vi "Connection_Management.vi"(0 "CM Packet In":T3, 5 "Commands":T7, 7 "Retry interval (ms)":i32, 9 "Number of tries":u8, 11 "error in (no error)":errorcluster) -> (4 "CM Packet Out":T3, 6 "CM Params Out":T2, 8 "Network Error Status":T1(ring), 15 "error out":errorcluster)   [LabVIEW 2017]
uses:
  Controls/Packet/Packet.ctl
  Controls/Packet/Packet_Direction.ctl
  Controls/Packet/Packet_Type.ctl
  Controls/Packet/Packet_Priority.ctl
  Controls/Connection Management/Connection_Management_Commands.ctl
  Controls/Control Packets/CM_Param.ctl
  <vilib>/Instr/_visa.llb/VISA Flush IO Buffer Mask.ctl
panel:
  out "Try counter (SYNC/RST)":i32
  out "Try counter (CC)":i32
  out "Try counter (OC)":i32
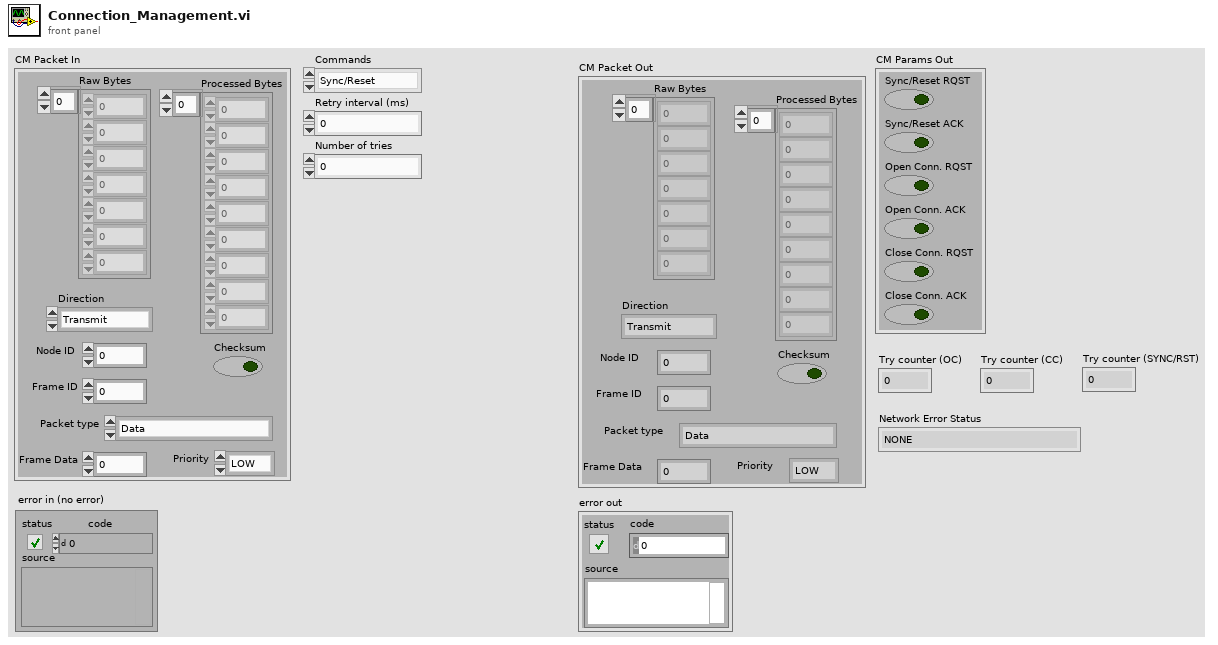
[diagram p1: front panel]
types:
  T1 = enum16{"NONE", "CONNECTION_ALREADY_OPEN", "CONNECTION_ALREADY_CLOSED", "INVALID_FRAME_REQUEST"}
  T2 = typedef "CM_Param.ctl" = cluster{"Sync/Reset RQST":bool, "Sync/Reset ACK":bool, "Open Conn. RQST":bool, "Open Conn. ACK":bool, "Close Conn. RQST":bool, "Close Conn. ACK":bool}
  T3 = typedef "Packet.ctl" = cluster{"Raw Bytes":u8[], "Checksum":bool, "Direction":T4, "Processed Bytes":u8[], "Node ID":u8, "Packet type":T5, "Frame Data":u32, "Priority":T6, "Frame ID":u8}
  T4 = typedef "Packet_Direction.ctl" = enum16{"Transmit", "Receive", "Bidirectional"}
  T5 = typedef "Packet_Type.ctl" = enum16{"Data", "Connection Management", "Remote Request", "Error/Status"}
  T6 = typedef "Packet_Priority.ctl" = enum16{"LOW", "HIGH"}
  T7 = typedef "Connection_Management_Commands.ctl" = enum16{"Sync/Reset", "Open Connection", "Close Connection"}
  T8 = typedef "VISA Flush IO Buffer Mask.ctl" = u16
  T9 = typedef "ES_Param.ctl" = cluster{"Status Request":bool, "Status Ack.":bool, "Receiver Queue Status":enum16{"OK", "EMPTY", "FULL"}, "Network Error Status":enum16{"NONE", "CONNECTION_ALREADY_OPEN", "CONNECTION_ALREADY_CLOSED", "INVALID_FRAME_REQUEST"}, "Application Error Code":u16, "Receiver Queue Size":i32}
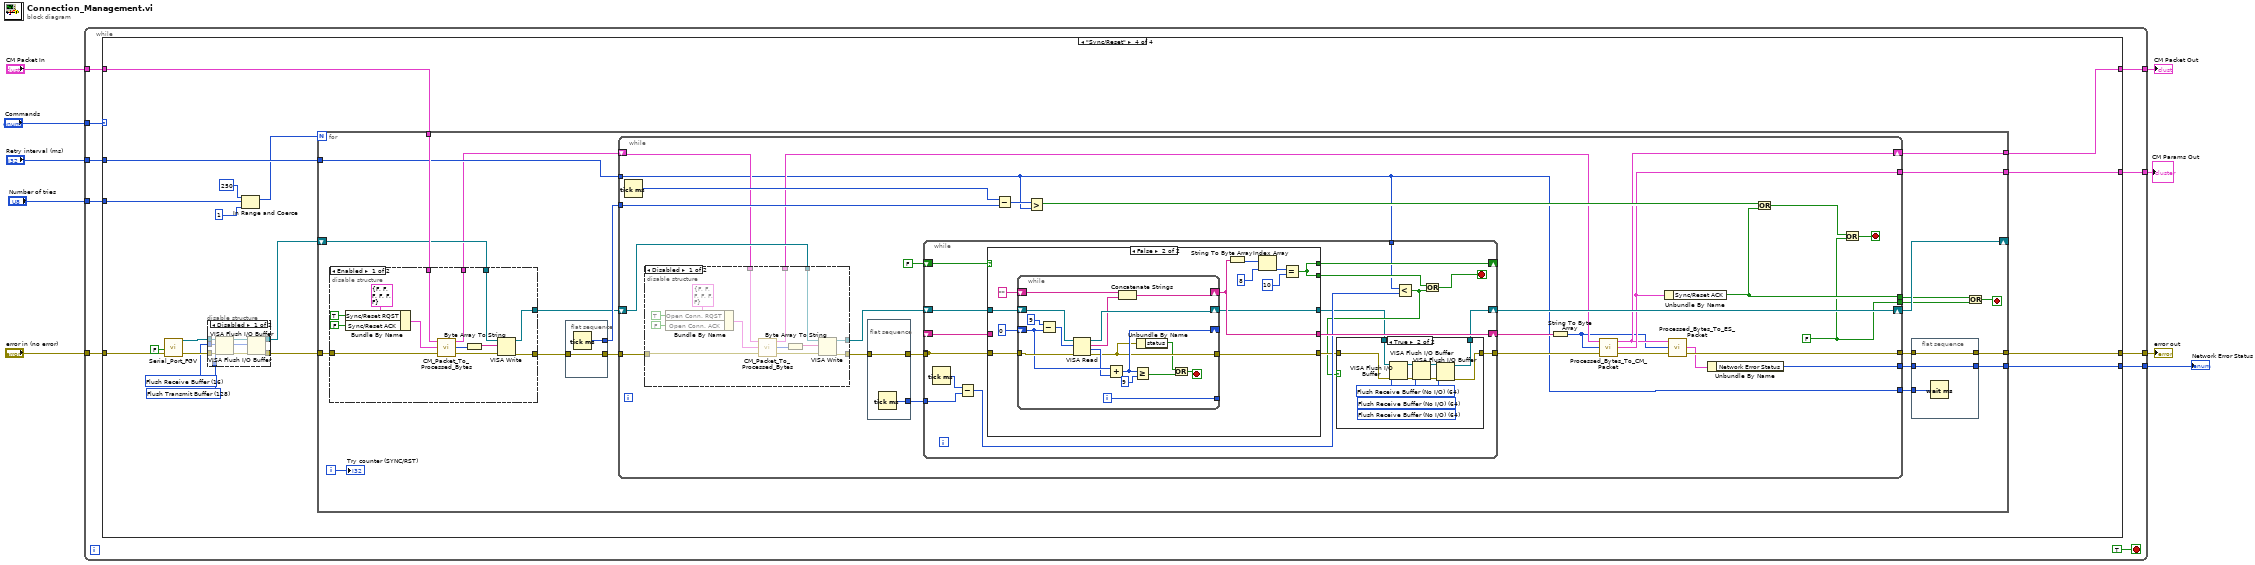
[diagram p0: block diagram]
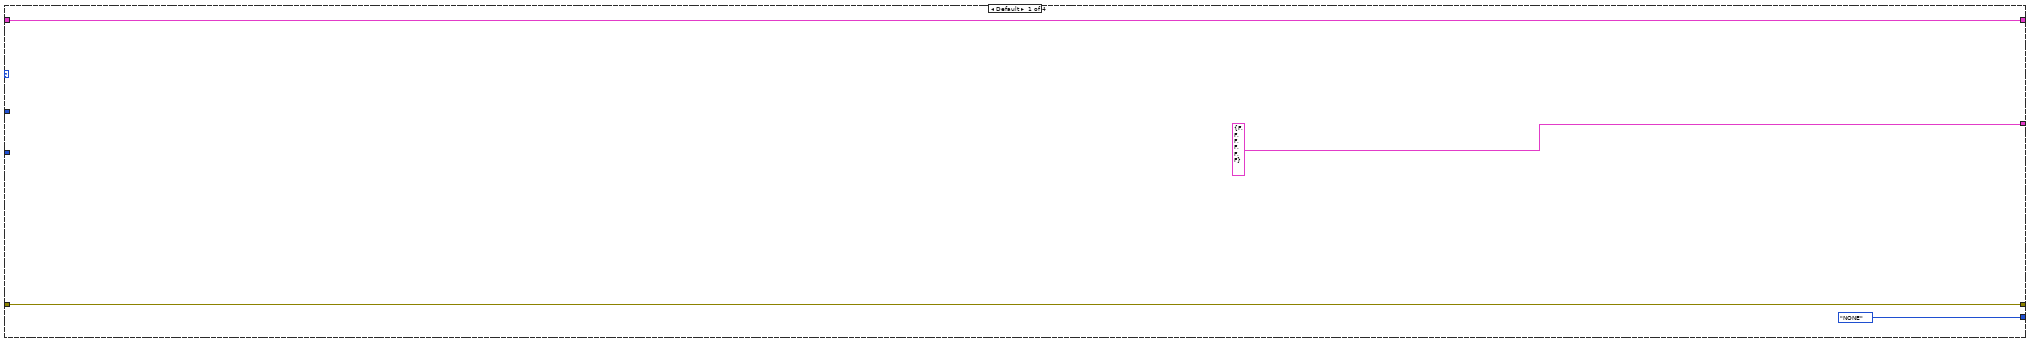
[diagram p2: hidden frame]
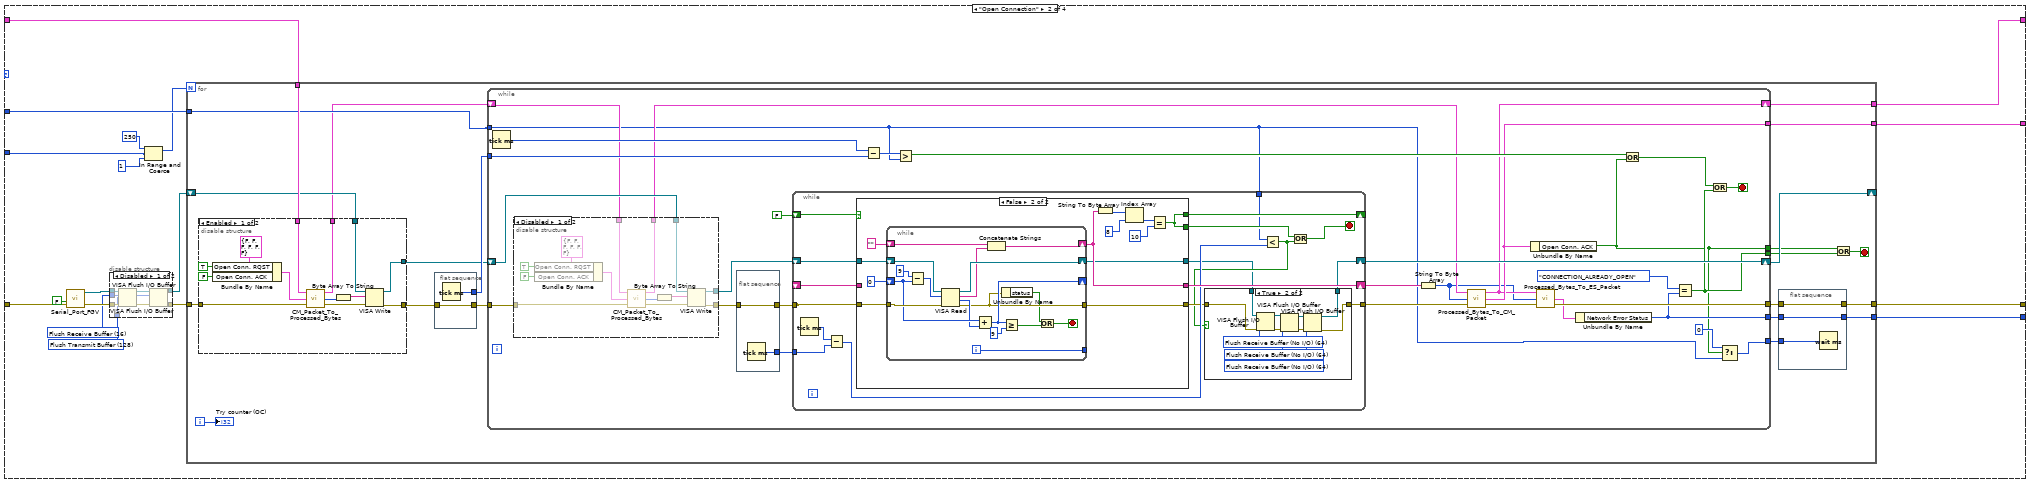
[diagram p3: hidden frame]
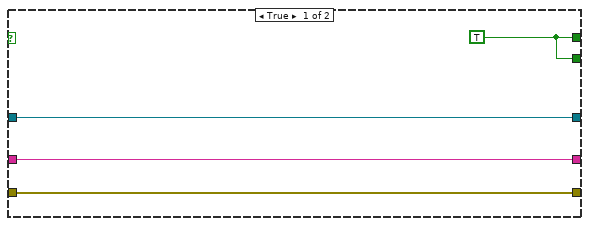
[diagram p8: hidden frame]
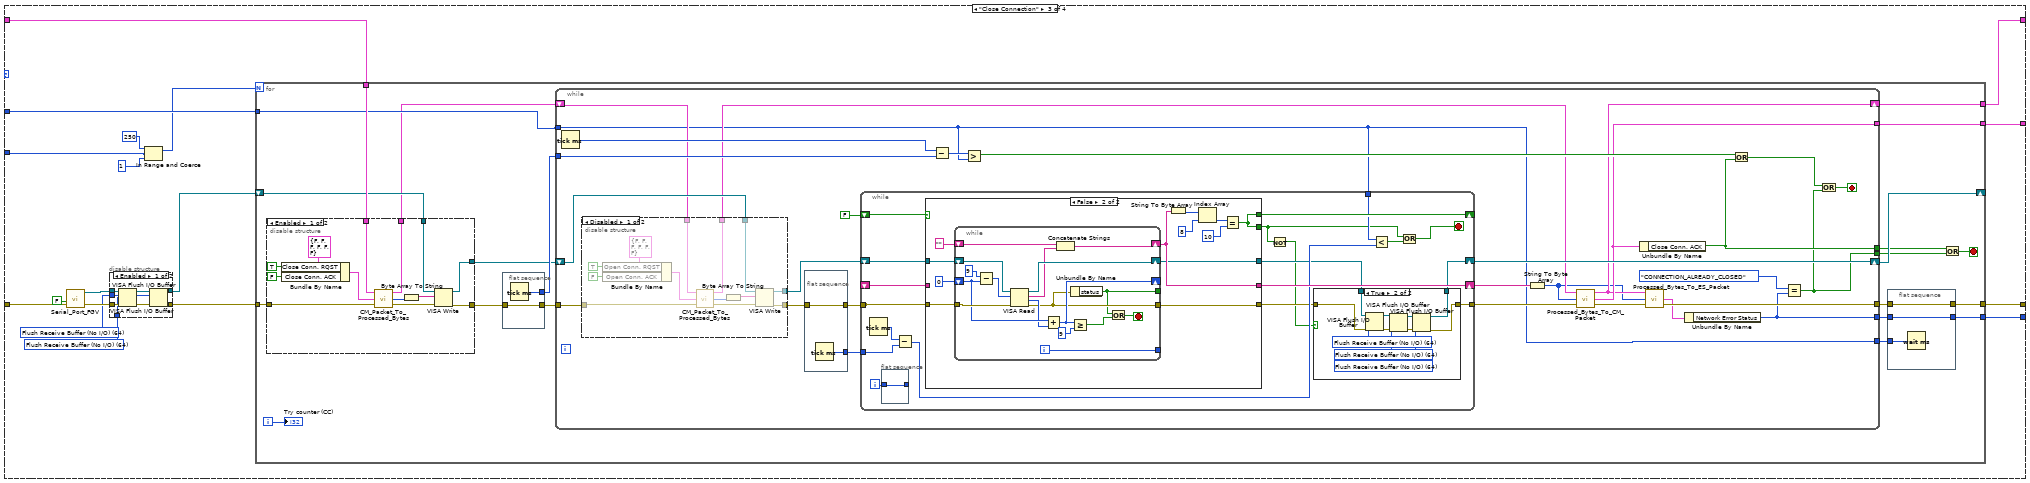
[diagram p9: hidden frame]
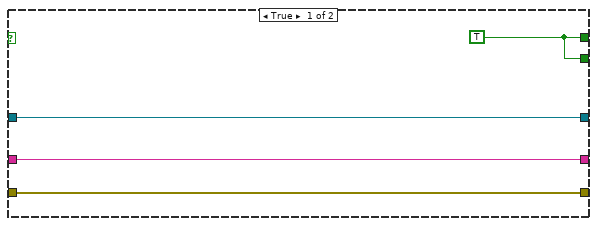
[diagram p14: hidden frame]
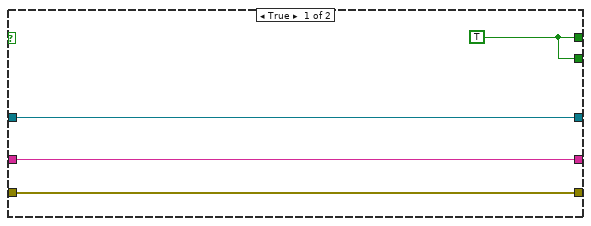
[diagram p19: hidden frame]
diagram:
  n1 = while {
    tunnel: "error in (no error)" -> [w18]
    tunnel: "Number of tries" -> [w13]
    tunnel: "Commands" -> [w17]
    tunnel: [w16] -> w4
    tunnel: "CM Packet In" -> [w15]
    tunnel: [w14] -> w5
    tunnel: "Retry interval (ms)" -> [w12]
    tunnel: [w11] -> w2
    tunnel: [w10] -> w1
    stop <- TRUE stop-if-true
    n2 = case shown="\"Sync/Reset\"" w17 {
      tunnel: w18 -> [w23 w38 w220 w403]
      tunnel: [w23 w33 w215 w398] -> w16
      tunnel: w15 -> [w22 w36 w218 w401]
      tunnel: [w22 w32 w214 w397] -> w14
      tunnel: w13 -> [_ w41 w223 w406]
      tunnel: w12 -> [_ w35 w217 w400]
      tunnel: [T2 {"Sync/Reset RQST"=FALSE, "Sync/Reset ACK"=FALSE, "Open Conn. RQST"=FALSE, "Open Conn. ACK"=FALSE, "Close Conn. RQST"=FALSE, "Close Conn. ACK"=FALSE} ("CM Params") w31 w213 w396] -> w11
      tunnel: [T1."NONE" ("Network Error Status") w24 w206 w389] -> w10
      frame Default {
      }
      frame "Open Connection" {
        w25 = T8 128 items=["Flush Receive Buffer"=16, "Write Transmit Buffer to Device"=32, "Flush Receive Buffer (No I/O)"=64, "Flush Transmit Buffer"=128] ("Mask")
        w26 = T8 16 items=["Flush Receive Buffer"=16, "Write Transmit Buffer to Device"=32, "Flush Receive Buffer (No I/O)"=64, "Flush Transmit Buffer"=128] ("Mask")
        n3 = call "Serial_Port_FGV.vi"("error in (no error)"=w38, "Initialize ?"=FALSE) -> ("error out"=w30:errorcluster, "COM Port out"=w28:refnum<visa-resource-name>)  [unwired: 8 in]
        n4 = disable-structure shown="Disabled" {
          disable-tunnel: w30 -> [w49 w50]
          disable-tunnel: [w47 w50] -> w29
          disable-tunnel: w28 -> [w46 w51]
          disable-tunnel: [w45 w51] -> w27
          disable-tunnel: w26 -> [w43 _]
          disable-tunnel: w25 -> [w42 _]
          frame Disabled {
            n5 = VISA Flush I/O Buffer(VISA resource name=w46, mask (16)=w43, error in (no error)=w49) -> (VISA resource name out=w44:refnum<visa-resource-name>, error out=w48:errorcluster)
            n6 = VISA Flush I/O Buffer(VISA resource name=w44, mask (16)=w42, error in (no error)=w48) -> (VISA resource name out=w45:refnum<visa-resource-name>, error out=w47:errorcluster)
          }
          frame Enabled {
          }
        }
        n7 = In Range and Coerce(upper limit=u8 250, x=w41, lower limit=u8 1) -> (coerced(x)=w34:u8)  [unwired: 1 out]
        n8 = for {
          N: w34 -> [_]
          tunnel: w29 -> [w72]
          tunnel: w36 -> [w71]
          shift-right: [w63] -> _
          shift-left: w27 -> [w70]
          tunnel: w35 -> [w67]
          tunnel: [w58] -> w33
          tunnel: [w62] -> w32
          tunnel: [w61] -> w31
          tunnel: [w52] -> w24
          i -> [w60]
          stop <- w56 stop-if-true
          n9 = disable-structure shown="Enabled" {
            disable-tunnel: w72 -> [w88 w89]
            disable-tunnel: w71 -> [w87 w91]
            disable-tunnel: w70 -> [w79 w90]
            disable-tunnel: [w78 w89] -> w69
            disable-tunnel: [w77 w90] -> w65
            disable-tunnel: [w76 w91] -> w64
            frame Enabled {
              n10 = Bundle By Name(cluster=T2 {"Sync/Reset RQST"=FALSE, "Sync/Reset ACK"=FALSE, "Open Conn. RQST"=FALSE, "Open Conn. ACK"=FALSE, "Close Conn. RQST"=FALSE, "Close Conn. ACK"=FALSE} ("Cluster"), "Open Conn. RQST"=TRUE, "Open Conn. ACK"=FALSE) -> (w84:T2)
              n11 = call "CM_Packet_To_Processed_Bytes.vi"("error in (no error)"=w88, "CM Params"=w84, "CM Packet In"=w87) -> ("error out"=w83:errorcluster, "Processed Bytes"=w81:u8[], "CM Packet Out"=w76:T3)
              n12 = Byte Array To String(unsigned byte array=w81) -> (string=w80:string)
              n13 = VISA Write(VISA resource name=w79, write buffer=w80, error in (no error)=w83) -> (VISA resource name out=w77:refnum<visa-resource-name>, error out=w78:errorcluster)  [unwired: 1 out]
            }
            frame Disabled {
            }
          }
          n14 = flat-sequence {
            tunnel: w69 -> [w205]
            tunnel: [w205] -> w68
            tunnel: [w204] -> w66
            frame #0 {
              n15 = Tick Count (ms)() -> (millisecond timer value=w204:u32)
            }
          }
          n16 = while {
            tunnel: w68 -> [w113]
            tunnel: w67 -> [w93]
            tunnel: w66 -> [w121]
            shift-right: [w116] -> w63
            shift-left: w65 -> [w112]
            shift-right: [w103] -> w62
            shift-left: w64 -> [w110]
            tunnel: [w104] -> w59
            tunnel: [w94] -> w55
            tunnel: [w114] -> w61
            tunnel: [w92] -> w57
            tunnel: [w100] -> w53
            tunnel: [w96] -> w54
            stop <- w97 stop-if-true
            n17 = Tick Count (ms)() -> (millisecond timer value=w122:u32)
            n18 = disable-structure shown="Disabled" {
              disable-tunnel: w113 -> [w130 w138]
              disable-tunnel: [w129 w138] -> w108
              disable-tunnel: w112 -> [w128 w139]
              disable-tunnel: [w127 w139] -> w111
              disable-tunnel: w110 -> [w126 w140]
              disable-tunnel: [w125 w140] -> w109
              frame Disabled {
                n19 = Bundle By Name(cluster=T2 {"Sync/Reset RQST"=FALSE, "Sync/Reset ACK"=FALSE, "Open Conn. RQST"=FALSE, "Open Conn. ACK"=FALSE, "Close Conn. RQST"=FALSE, "Close Conn. ACK"=FALSE} ("Cluster"), "Open Conn. RQST"=TRUE, "Open Conn. ACK"=FALSE) -> (w135:T2)
                n20 = call "CM_Packet_To_Processed_Bytes.vi"("error in (no error)"=w130, "CM Params"=w135, "CM Packet In"=w126) -> ("error out"=w134:errorcluster, "Processed Bytes"=w132:u8[], "CM Packet Out"=w125:T3)
                n21 = Byte Array To String(unsigned byte array=w132) -> (string=w131:string)
                n22 = VISA Write(VISA resource name=w128, write buffer=w131, error in (no error)=w134) -> (VISA resource name out=w127:refnum<visa-resource-name>, error out=w129:errorcluster)  [unwired: 1 out]
              }
              frame Enabled {
              }
            }
            n23 = flat-sequence {
              tunnel: w108 -> [w124]
              tunnel: [w124] -> w107
              tunnel: [w123] -> w106
              frame #0 {
                n24 = Tick Count (ms)() -> (millisecond timer value=w123:u32)
              }
            }
            n25 = while {
              tunnel: [w151] -> _
              shift-right: [w155] -> _
              shift-left: FALSE -> [w156]
              tunnel: [w145] -> w117
              shift-right: [w154] -> w118
              shift-left: _ -> [w153]
              shift-right: [w142] -> w116
              shift-left: w111 -> [w157]
              tunnel: w107 -> [w151]
              tunnel: w106 -> [w149]
              tunnel: w93 -> [w147]
              stop <- w141 stop-if-true
              n26 = Tick Count (ms)() -> (millisecond timer value=w150:u32)
              n27 = Subtract(x=w150, y=w149) -> (x-y=w148:u32)
              n28 = case shown="False" w156 {
                tunnel: w151 -> [w173 w186]
                tunnel: w157 -> [w171 w184]
                tunnel: [w174 w178] -> w152
                tunnel: [w174 w178] -> w155
                tunnel: [w173 w177] -> w146
                tunnel: [w172 w176] -> w154
                tunnel: w153 -> [w172 _]
                tunnel: [w171 w175] -> w143
                frame True {
                  w174 = TRUE
                }
                frame False {
                  n29 = while {
                    tunnel: w186 -> [w203]
                    shift-right: [w193] -> _
                    shift-left: 0 -> [w196]
                    shift-right: [w199] -> w175
                    shift-left: w184 -> [w200]
                    shift-right: [w192] -> w176
                    shift-left: "" -> [w198]
                    tunnel: [w188] -> w177
                    tunnel: [w191] -> _
                    i -> [w191]
                    stop <- w190 stop-if-true
                    n30 = Subtract(x=9, y=w196) -> (x-y=w201:u32)
                    n31 = VISA Read(VISA resource name=w200, byte count=w201, error in (no error)=w203) -> (VISA resource name out=w199:refnum<visa-resource-name>, read buffer=w197:string, return count=w195:u32, error out=w188:errorcluster)
                    n32 = Add(x=w196, y=w195) -> (x+y=w193:u32)
                    n33 = Concatenate Strings(w198, w197) -> (w192:string)
                    n34 = Unbundle By Name(w188) -> ("status"=w187:bool)
                    n35 = Greater Or Equal?(x=w193, y=u32 9) -> (x >= y?=w189:bool)
                    n36 = Or(x=w187, y=w189) -> (x .or. y?=w190:bool)
                  }
                  n37 = String To Byte Array(string=w176) -> (unsigned byte array=w182:u8[])
                  n38 = Index Array(array=w182, index=8) -> (element=w180:u8)
                  n39 = Equal?(x=w180, y=u8 10) -> (x = y?=w178:bool)
                }
              }
              n40 = Less?(x=w147, y=w148) -> (x < y?=w144:bool)
              n41 = case shown="True" w144 {
                tunnel: w146 -> [w159 w170]
                tunnel: [w159 w167] -> w145
                tunnel: w143 -> [w158 w166]
                tunnel: [w158 w163] -> w142
                frame False {
                }
                frame True {
                  w160 = T8 64 items=["Flush Receive Buffer"=16, "Write Transmit Buffer to Device"=32, "Flush Receive Buffer (No I/O)"=64, "Flush Transmit Buffer"=128] ("Mask")
                  w161 = T8 64 items=["Flush Receive Buffer"=16, "Write Transmit Buffer to Device"=32, "Flush Receive Buffer (No I/O)"=64, "Flush Transmit Buffer"=128] ("Mask")
                  w162 = T8 64 items=["Flush Receive Buffer"=16, "Write Transmit Buffer to Device"=32, "Flush Receive Buffer (No I/O)"=64, "Flush Transmit Buffer"=128] ("Mask")
                  n42 = VISA Flush I/O Buffer(VISA resource name=w166, mask (16)=w162, error in (no error)=w170) -> (VISA resource name out=w165:refnum<visa-resource-name>, error out=w169:errorcluster)
                  n43 = VISA Flush I/O Buffer(VISA resource name=w165, mask (16)=w161, error in (no error)=w169) -> (VISA resource name out=w164:refnum<visa-resource-name>, error out=w168:errorcluster)
                  n44 = VISA Flush I/O Buffer(VISA resource name=w164, mask (16)=w160, error in (no error)=w168) -> (VISA resource name out=w163:refnum<visa-resource-name>, error out=w167:errorcluster)
                }
              }
              n45 = Or(x=w152, y=w144) -> (x .or. y?=w141:bool)
            }
            n46 = Subtract(x=w122, y=w121) -> (x-y=w120:u32)
            n47 = Greater?(x=w120, y=w93) -> (0:w115:bool)
            n48 = String To Byte Array(string=w118) -> (unsigned byte array=w102:u8[])
            n49 = call "Processed_Bytes_To_CM_Packet.vi"("error in (no error)"=w117, "Processed Byte"=w102, "CM Packet In"=w109) -> ("error out"=w105:errorcluster, "CM Params"=w114:T2, "CM Packet Out"=w103:T3)
            n50 = Unbundle By Name(w114) -> ("Open Conn. ACK"=w94:bool)
            n51 = call "Processed_Bytes_To_ES_Packet.vi"("error in (no error)"=w105, "Processed_Bytes"=w102, "ES Packet In"=w103) -> ("error out"=w104:errorcluster, "ES Param Out"=w101:T9)  [unwired: 1 out]
            n52 = Unbundle By Name(w101) -> ("Network Error Status"=w100:T1)
            n53 = Or(x=w115, y=w94) -> (x .or. y?=w98:bool)
            n54 = Equal?(x=T1."CONNECTION_ALREADY_OPEN", y=w100) -> (x = y?=w96:bool)
            n55 = Or(x=w98, y=w96) -> (x .or. y?=w97:bool)
            n56 = Select(t=0, s=w94, f=w93) -> (s? t:f=w92:i32)
          }
          n57 = flat-sequence {
            tunnel: w59 -> [w75]
            tunnel: [w75] -> w58
            tunnel: w57 -> [w74]
            tunnel: w53 -> [w73]
            tunnel: [w73] -> w52
            frame #0 {
              n58 = Wait (ms)(milliseconds to wait=w74) -> ()  [unwired: 1 out]
            }
          }
          n59 = Or(x=w55, y=w54) -> (x .or. y?=w56:bool)
          "Try counter (OC)" <- w60
        }
      }
      frame "Close Connection" {
        w207 = T8 64 items=["Flush Receive Buffer"=16, "Write Transmit Buffer to Device"=32, "Flush Receive Buffer (No I/O)"=64, "Flush Transmit Buffer"=128] ("Mask")
        w208 = T8 64 items=["Flush Receive Buffer"=16, "Write Transmit Buffer to Device"=32, "Flush Receive Buffer (No I/O)"=64, "Flush Transmit Buffer"=128] ("Mask")
        n60 = call "Serial_Port_FGV.vi"("error in (no error)"=w220, "Initialize ?"=FALSE) -> ("error out"=w212:errorcluster, "COM Port out"=w210:refnum<visa-resource-name>)  [unwired: 8 in]
        n61 = disable-structure shown="Enabled" {
          disable-tunnel: w212 -> [w231 w232]
          disable-tunnel: [w229 w232] -> w211
          disable-tunnel: w210 -> [w228 w233]
          disable-tunnel: [w227 w233] -> w209
          disable-tunnel: w208 -> [w225 _]
          disable-tunnel: w207 -> [w224 _]
          frame Enabled {
            n62 = VISA Flush I/O Buffer(VISA resource name=w228, mask (16)=w225, error in (no error)=w231) -> (VISA resource name out=w226:refnum<visa-resource-name>, error out=w230:errorcluster)
            n63 = VISA Flush I/O Buffer(VISA resource name=w226, mask (16)=w224, error in (no error)=w230) -> (VISA resource name out=w227:refnum<visa-resource-name>, error out=w229:errorcluster)
          }
          frame Disabled {
          }
        }
        n64 = In Range and Coerce(upper limit=u8 250, x=w223, lower limit=u8 1) -> (coerced(x)=w216:u8)  [unwired: 1 out]
        n65 = for {
          N: w216 -> [_]
          tunnel: w211 -> [w254]
          tunnel: w218 -> [w253]
          shift-right: [w245] -> _
          shift-left: w209 -> [w252]
          tunnel: w217 -> [w249]
          tunnel: [w240] -> w215
          tunnel: [w244] -> w214
          tunnel: [w243] -> w213
          tunnel: [w234] -> w206
          i -> [w242]
          stop <- w238 stop-if-true
          n66 = disable-structure shown="Enabled" {
            disable-tunnel: w254 -> [w270 w271]
            disable-tunnel: w253 -> [w269 w273]
            disable-tunnel: w252 -> [w261 w272]
            disable-tunnel: [w260 w271] -> w251
            disable-tunnel: [w259 w272] -> w247
            disable-tunnel: [w258 w273] -> w246
            frame Enabled {
              n67 = Bundle By Name(cluster=T2 {"Sync/Reset RQST"=FALSE, "Sync/Reset ACK"=FALSE, "Open Conn. RQST"=FALSE, "Open Conn. ACK"=FALSE, "Close Conn. RQST"=FALSE, "Close Conn. ACK"=FALSE} ("Cluster"), "Close Conn. RQST"=TRUE ("Open Conn. RQST"), "Close Conn. ACK"=FALSE ("Open Conn. ACK")) -> (w266:T2)
              n68 = call "CM_Packet_To_Processed_Bytes.vi"("error in (no error)"=w270, "CM Params"=w266, "CM Packet In"=w269) -> ("error out"=w265:errorcluster, "Processed Bytes"=w263:u8[], "CM Packet Out"=w258:T3)
              n69 = Byte Array To String(unsigned byte array=w263) -> (string=w262:string)
              n70 = VISA Write(VISA resource name=w261, write buffer=w262, error in (no error)=w265) -> (VISA resource name out=w259:refnum<visa-resource-name>, error out=w260:errorcluster)  [unwired: 1 out]
            }
            frame Disabled {
            }
          }
          n71 = flat-sequence {
            tunnel: w251 -> [w388]
            tunnel: [w388] -> w250
            tunnel: [w387] -> w248
            frame #0 {
              n72 = Tick Count (ms)() -> (millisecond timer value=w387:u32)
            }
          }
          n73 = while {
            tunnel: w250 -> [w292]
            tunnel: w249 -> [w284]
            tunnel: w248 -> [w301]
            shift-right: [w296] -> w245
            shift-left: w247 -> [w291]
            shift-right: [w281] -> w244
            shift-left: w246 -> [w289]
            tunnel: [w282] -> w241
            tunnel: [w294] -> w237
            tunnel: [w293] -> w243
            tunnel: [w284] -> w239
            tunnel: [w278] -> w235
            tunnel: [w274] -> w236
            stop <- w275 stop-if-true
            n74 = Tick Count (ms)() -> (millisecond timer value=w302:u32)
            n75 = disable-structure shown="Disabled" {
              disable-tunnel: w292 -> [w310 w318]
              disable-tunnel: [w309 w318] -> w287
              disable-tunnel: w291 -> [w308 w319]
              disable-tunnel: [w307 w319] -> w290
              disable-tunnel: w289 -> [w306 w320]
              disable-tunnel: [w305 w320] -> w288
              frame Disabled {
                n76 = Bundle By Name(cluster=T2 {"Sync/Reset RQST"=FALSE, "Sync/Reset ACK"=FALSE, "Open Conn. RQST"=FALSE, "Open Conn. ACK"=FALSE, "Close Conn. RQST"=FALSE, "Close Conn. ACK"=FALSE} ("Cluster"), "Open Conn. RQST"=TRUE, "Open Conn. ACK"=FALSE) -> (w315:T2)
                n77 = call "CM_Packet_To_Processed_Bytes.vi"("error in (no error)"=w310, "CM Params"=w315, "CM Packet In"=w306) -> ("error out"=w314:errorcluster, "Processed Bytes"=w312:u8[], "CM Packet Out"=w305:T3)
                n78 = Byte Array To String(unsigned byte array=w312) -> (string=w311:string)
                n79 = VISA Write(VISA resource name=w308, write buffer=w311, error in (no error)=w314) -> (VISA resource name out=w307:refnum<visa-resource-name>, error out=w309:errorcluster)  [unwired: 1 out]
              }
              frame Enabled {
              }
            }
            n80 = flat-sequence {
              tunnel: w287 -> [w304]
              tunnel: [w304] -> w286
              tunnel: [w303] -> w285
              frame #0 {
                n81 = Tick Count (ms)() -> (millisecond timer value=w303:u32)
              }
            }
            n82 = while {
              tunnel: [w334] -> _
              shift-right: [w337] -> _
              shift-left: FALSE -> [w338]
              tunnel: [w328] -> w297
              shift-right: [w336] -> w298
              shift-left: _ -> [w335]
              shift-right: [w325] -> w296
              shift-left: w290 -> [w339]
              tunnel: w286 -> [w334]
              tunnel: w285 -> [w332]
              tunnel: w284 -> [w330]
              i -> [w324]
              stop <- w323 stop-if-true
              n83 = Tick Count (ms)() -> (millisecond timer value=w333:u32)
              n84 = flat-sequence {
                tunnel: w324 -> [w340]
                tunnel: [w340] -> _
                frame #0 {
                }
              }
              n85 = Subtract(x=w333, y=w332) -> (x-y=w331:u32)
              n86 = case shown="False" w338 {
                tunnel: w334 -> [w356 w369]
                tunnel: w339 -> [w354 w367]
                tunnel: [w357 w361] -> w322
                tunnel: [w357 w361] -> w337
                tunnel: [w356 w360] -> w329
                tunnel: [w355 w359] -> w336
                tunnel: w335 -> [w355 _]
                tunnel: [w354 w358] -> w326
                frame True {
                  w357 = TRUE
                }
                frame False {
                  n87 = while {
                    tunnel: w369 -> [w386]
                    shift-right: [w376] -> _
                    shift-left: 0 -> [w379]
                    shift-right: [w382] -> w358
                    shift-left: w367 -> [w383]
                    shift-right: [w375] -> w359
                    shift-left: "" -> [w381]
                    tunnel: [w373] -> w360
                    tunnel: [w374] -> _
                    tunnel: [w370] -> _
                    i -> [w374]
                    stop <- w372 stop-if-true
                    n88 = Subtract(x=9, y=w379) -> (x-y=w384:u32)
                    n89 = VISA Read(VISA resource name=w383, byte count=w384, error in (no error)=w386) -> (VISA resource name out=w382:refnum<visa-resource-name>, read buffer=w380:string, return count=w378:u32, error out=w373:errorcluster)
                    n90 = Add(x=w379, y=w378) -> (x+y=w376:u32)
                    n91 = Concatenate Strings(w381, w380) -> (w375:string)
                    n92 = Unbundle By Name(w373) -> ("status"=w370:bool)
                    n93 = Greater Or Equal?(x=w376, y=u32 9) -> (x >= y?=w371:bool)
                    n94 = Or(x=w370, y=w371) -> (x .or. y?=w372:bool)
                  }
                  n95 = String To Byte Array(string=w359) -> (unsigned byte array=w365:u8[])
                  n96 = Index Array(array=w365, index=8) -> (element=w363:u8)
                  n97 = Equal?(x=w363, y=u8 10) -> (x = y?=w361:bool)
                }
              }
              n98 = Not(x=w322) -> (.not. x?=w321:bool)
              n99 = case shown="True" w321 {
                tunnel: w329 -> [w342 w353]
                tunnel: [w342 w350] -> w328
                tunnel: w326 -> [w341 w349]
                tunnel: [w341 w346] -> w325
                frame False {
                }
                frame True {
                  w343 = T8 64 items=["Flush Receive Buffer"=16, "Write Transmit Buffer to Device"=32, "Flush Receive Buffer (No I/O)"=64, "Flush Transmit Buffer"=128] ("Mask")
                  w344 = T8 64 items=["Flush Receive Buffer"=16, "Write Transmit Buffer to Device"=32, "Flush Receive Buffer (No I/O)"=64, "Flush Transmit Buffer"=128] ("Mask")
                  w345 = T8 64 items=["Flush Receive Buffer"=16, "Write Transmit Buffer to Device"=32, "Flush Receive Buffer (No I/O)"=64, "Flush Transmit Buffer"=128] ("Mask")
                  n100 = VISA Flush I/O Buffer(VISA resource name=w349, mask (16)=w345, error in (no error)=w353) -> (VISA resource name out=w348:refnum<visa-resource-name>, error out=w352:errorcluster)
                  n101 = VISA Flush I/O Buffer(VISA resource name=w348, mask (16)=w344, error in (no error)=w352) -> (VISA resource name out=w347:refnum<visa-resource-name>, error out=w351:errorcluster)
                  n102 = VISA Flush I/O Buffer(VISA resource name=w347, mask (16)=w343, error in (no error)=w351) -> (VISA resource name out=w346:refnum<visa-resource-name>, error out=w350:errorcluster)
                }
              }
              n103 = Less?(x=w330, y=w331) -> (x < y?=w327:bool)
              n104 = Or(x=w322, y=w327) -> (x .or. y?=w323:bool)
            }
            n105 = Subtract(x=w302, y=w301) -> (x-y=w300:u32)
            n106 = Greater?(x=w300, y=w284) -> (0:w295:bool)
            n107 = String To Byte Array(string=w298) -> (unsigned byte array=w280:u8[])
            n108 = call "Processed_Bytes_To_CM_Packet.vi"("error in (no error)"=w297, "Processed Byte"=w280, "CM Packet In"=w288) -> ("error out"=w283:errorcluster, "CM Params"=w293:T2, "CM Packet Out"=w281:T3)
            n109 = Unbundle By Name(w293) -> ("Close Conn. ACK"=w294:bool)
            n110 = call "Processed_Bytes_To_ES_Packet.vi"("error in (no error)"=w283, "Processed_Bytes"=w280, "ES Packet In"=w281) -> ("error out"=w282:errorcluster, "ES Param Out"=w279:T9)  [unwired: 1 out]
            n111 = Unbundle By Name(w279) -> ("Network Error Status"=w278:T1)
            n112 = Or(x=w295, y=w294) -> (x .or. y?=w276:bool)
            n113 = Equal?(x=T1."CONNECTION_ALREADY_CLOSED", y=w278) -> (x = y?=w274:bool)
            n114 = Or(x=w276, y=w274) -> (x .or. y?=w275:bool)
          }
          n115 = flat-sequence {
            tunnel: w241 -> [w257]
            tunnel: [w257] -> w240
            tunnel: w239 -> [w256]
            tunnel: w235 -> [w255]
            tunnel: [w255] -> w234
            frame #0 {
              n116 = Wait (ms)(milliseconds to wait=w256) -> ()  [unwired: 1 out]
            }
          }
          n117 = Or(x=w237, y=w236) -> (x .or. y?=w238:bool)
          "Try counter (CC)" <- w242
        }
      }
      frame "Sync/Reset" {
        w390 = T8 128 items=["Flush Receive Buffer"=16, "Write Transmit Buffer to Device"=32, "Flush Receive Buffer (No I/O)"=64, "Flush Transmit Buffer"=128] ("Mask")
        w391 = T8 16 items=["Flush Receive Buffer"=16, "Write Transmit Buffer to Device"=32, "Flush Receive Buffer (No I/O)"=64, "Flush Transmit Buffer"=128] ("Mask")
        n118 = call "Serial_Port_FGV.vi"("error in (no error)"=w403, "Initialize ?"=FALSE) -> ("error out"=w395:errorcluster, "COM Port out"=w393:refnum<visa-resource-name>)  [unwired: 8 in]
        n119 = disable-structure shown="Disabled" {
          disable-tunnel: w395 -> [w414 w415]
          disable-tunnel: [w412 w415] -> w394
          disable-tunnel: w393 -> [w411 w416]
          disable-tunnel: [w410 w416] -> w392
          disable-tunnel: w391 -> [w408 _]
          disable-tunnel: w390 -> [w407 _]
          frame Disabled {
            n120 = VISA Flush I/O Buffer(VISA resource name=w411, mask (16)=w408, error in (no error)=w414) -> (VISA resource name out=w409:refnum<visa-resource-name>, error out=w413:errorcluster)
            n121 = VISA Flush I/O Buffer(VISA resource name=w409, mask (16)=w407, error in (no error)=w413) -> (VISA resource name out=w410:refnum<visa-resource-name>, error out=w412:errorcluster)
          }
          frame Enabled {
          }
        }
        n122 = In Range and Coerce(upper limit=u8 250, x=w406, lower limit=u8 1) -> (coerced(x)=w399:u8)  [unwired: 1 out]
        n123 = for {
          N: w399 -> [_]
          tunnel: w394 -> [w437]
          tunnel: w401 -> [w436]
          shift-right: [w428] -> _
          shift-left: w392 -> [w435]
          tunnel: w400 -> [w432]
          tunnel: [w423] -> w398
          tunnel: [w427] -> w397
          tunnel: [w426] -> w396
          tunnel: [w417] -> w389
          i -> [w425]
          stop <- w421 stop-if-true
          n124 = disable-structure shown="Enabled" {
            disable-tunnel: w437 -> [w453 w454]
            disable-tunnel: w436 -> [w452 w456]
            disable-tunnel: w435 -> [w445 w455]
            disable-tunnel: [w444 w454] -> w434
            disable-tunnel: [w443 w455] -> w430
            disable-tunnel: [w442 w456] -> w429
            frame Enabled {
              n125 = Bundle By Name(cluster=T2 {"Sync/Reset RQST"=FALSE, "Sync/Reset ACK"=FALSE, "Open Conn. RQST"=FALSE, "Open Conn. ACK"=FALSE, "Close Conn. RQST"=FALSE, "Close Conn. ACK"=FALSE} ("Cluster"), "Sync/Reset RQST"=TRUE ("Open Conn. RQST"), "Sync/Reset ACK"=FALSE ("Open Conn. ACK")) -> (w449:T2)
              n126 = call "CM_Packet_To_Processed_Bytes.vi"("error in (no error)"=w453, "CM Params"=w449, "CM Packet In"=w452) -> ("error out"=w441:errorcluster, "Processed Bytes"=w447:u8[], "CM Packet Out"=w442:T3)
              n127 = Byte Array To String(unsigned byte array=w447) -> (string=w446:string)
              n128 = VISA Write(VISA resource name=w445, write buffer=w446, error in (no error)=w441) -> (VISA resource name out=w443:refnum<visa-resource-name>, error out=w444:errorcluster)  [unwired: 1 out]
            }
            frame Disabled {
            }
          }
          n129 = flat-sequence {
            tunnel: w434 -> [w567]
            tunnel: [w567] -> w433
            tunnel: [w566] -> w431
            frame #0 {
              n130 = Tick Count (ms)() -> (millisecond timer value=w566:u32)
            }
          }
          n131 = while {
            tunnel: w433 -> [w474]
            tunnel: w432 -> [w466]
            tunnel: w431 -> [w483]
            shift-right: [w478] -> w428
            shift-left: w430 -> [w473]
            shift-right: [w463] -> w427
            shift-left: w429 -> [w471]
            tunnel: [w464] -> w424
            tunnel: [w476] -> w420
            tunnel: [w475] -> w426
            tunnel: [w466] -> w422
            tunnel: [w460] -> w418
            tunnel: [w457] -> w419
            stop <- w458 stop-if-true
            w457 = FALSE
            n132 = Tick Count (ms)() -> (millisecond timer value=w484:u32)
            n133 = disable-structure shown="Disabled" {
              disable-tunnel: w474 -> [w492 w500]
              disable-tunnel: [w491 w500] -> w469
              disable-tunnel: w473 -> [w490 w501]
              disable-tunnel: [w489 w501] -> w472
              disable-tunnel: w471 -> [w488 w502]
              disable-tunnel: [w487 w502] -> w470
              frame Disabled {
                n134 = Bundle By Name(cluster=T2 {"Sync/Reset RQST"=FALSE, "Sync/Reset ACK"=FALSE, "Open Conn. RQST"=FALSE, "Open Conn. ACK"=FALSE, "Close Conn. RQST"=FALSE, "Close Conn. ACK"=FALSE} ("Cluster"), "Open Conn. RQST"=TRUE, "Open Conn. ACK"=FALSE) -> (w497:T2)
                n135 = call "CM_Packet_To_Processed_Bytes.vi"("error in (no error)"=w492, "CM Params"=w497, "CM Packet In"=w488) -> ("error out"=w496:errorcluster, "Processed Bytes"=w494:u8[], "CM Packet Out"=w487:T3)
                n136 = Byte Array To String(unsigned byte array=w494) -> (string=w493:string)
                n137 = VISA Write(VISA resource name=w490, write buffer=w493, error in (no error)=w496) -> (VISA resource name out=w489:refnum<visa-resource-name>, error out=w491:errorcluster)  [unwired: 1 out]
              }
              frame Enabled {
              }
            }
            n138 = flat-sequence {
              tunnel: w469 -> [w486]
              tunnel: [w486] -> w468
              tunnel: [w485] -> w467
              frame #0 {
                n139 = Tick Count (ms)() -> (millisecond timer value=w485:u32)
              }
            }
            n140 = while {
              tunnel: [w513] -> _
              shift-right: [w517] -> _
              shift-left: FALSE -> [w518]
              tunnel: [w507] -> w479
              shift-right: [w516] -> w480
              shift-left: _ -> [w515]
              shift-right: [w504] -> w478
              shift-left: w472 -> [w519]
              tunnel: w468 -> [w513]
              tunnel: w467 -> [w511]
              tunnel: w466 -> [w509]
              stop <- w503 stop-if-true
              n141 = Tick Count (ms)() -> (millisecond timer value=w512:u32)
              n142 = Subtract(x=w512, y=w511) -> (x-y=w510:u32)
              n143 = case shown="False" w518 {
                tunnel: w513 -> [w535 w548]
                tunnel: w519 -> [w533 w546]
                tunnel: [w536 w540] -> w514
                tunnel: [w536 w540] -> w517
                tunnel: [w535 w539] -> w508
                tunnel: [w534 w538] -> w516
                tunnel: w515 -> [w534 _]
                tunnel: [w533 w537] -> w505
                frame True {
                  w536 = TRUE
                }
                frame False {
                  n144 = while {
                    tunnel: w548 -> [w565]
                    shift-right: [w555] -> _
                    shift-left: 0 -> [w558]
                    shift-right: [w561] -> w537
                    shift-left: w546 -> [w562]
                    shift-right: [w554] -> w538
                    shift-left: "" -> [w560]
                    tunnel: [w550] -> w539
                    tunnel: [w553] -> _
                    i -> [w553]
                    stop <- w552 stop-if-true
                    n145 = Subtract(x=9, y=w558) -> (x-y=w563:u32)
                    n146 = VISA Read(VISA resource name=w562, byte count=w563, error in (no error)=w565) -> (VISA resource name out=w561:refnum<visa-resource-name>, read buffer=w559:string, return count=w557:u32, error out=w550:errorcluster)
                    n147 = Add(x=w558, y=w557) -> (x+y=w555:u32)
                    n148 = Concatenate Strings(w560, w559) -> (w554:string)
                    n149 = Greater Or Equal?(x=w555, y=u32 9) -> (x >= y?=w551:bool)
                    n150 = Unbundle By Name(w550) -> ("status"=w549:bool)
                    n151 = Or(x=w549, y=w551) -> (x .or. y?=w552:bool)
                  }
                  n152 = String To Byte Array(string=w538) -> (unsigned byte array=w544:u8[])
                  n153 = Index Array(array=w544, index=8) -> (element=w542:u8)
                  n154 = Equal?(x=w542, y=u8 10) -> (x = y?=w540:bool)
                }
              }
              n155 = Less?(x=w509, y=w510) -> (x < y?=w506:bool)
              n156 = case shown="True" w506 {
                tunnel: w508 -> [w521 w532]
                tunnel: [w521 w529] -> w507
                tunnel: w505 -> [w520 w528]
                tunnel: [w520 w525] -> w504
                frame False {
                }
                frame True {
                  w522 = T8 64 items=["Flush Receive Buffer"=16, "Write Transmit Buffer to Device"=32, "Flush Receive Buffer (No I/O)"=64, "Flush Transmit Buffer"=128] ("Mask")
                  w523 = T8 64 items=["Flush Receive Buffer"=16, "Write Transmit Buffer to Device"=32, "Flush Receive Buffer (No I/O)"=64, "Flush Transmit Buffer"=128] ("Mask")
                  w524 = T8 64 items=["Flush Receive Buffer"=16, "Write Transmit Buffer to Device"=32, "Flush Receive Buffer (No I/O)"=64, "Flush Transmit Buffer"=128] ("Mask")
                  n157 = VISA Flush I/O Buffer(VISA resource name=w528, mask (16)=w524, error in (no error)=w532) -> (VISA resource name out=w527:refnum<visa-resource-name>, error out=w531:errorcluster)
                  n158 = VISA Flush I/O Buffer(VISA resource name=w527, mask (16)=w523, error in (no error)=w531) -> (VISA resource name out=w526:refnum<visa-resource-name>, error out=w530:errorcluster)
                  n159 = VISA Flush I/O Buffer(VISA resource name=w526, mask (16)=w522, error in (no error)=w530) -> (VISA resource name out=w525:refnum<visa-resource-name>, error out=w529:errorcluster)
                }
              }
              n160 = Or(x=w514, y=w506) -> (x .or. y?=w503:bool)
            }
            n161 = Subtract(x=w484, y=w483) -> (x-y=w482:u32)
            n162 = Greater?(x=w482, y=w466) -> (0:w477:bool)
            n163 = String To Byte Array(string=w480) -> (unsigned byte array=w462:u8[])
            n164 = call "Processed_Bytes_To_CM_Packet.vi"("error in (no error)"=w479, "Processed Byte"=w462, "CM Packet In"=w470) -> ("error out"=w465:errorcluster, "CM Params"=w475:T2, "CM Packet Out"=w463:T3)
            n165 = Unbundle By Name(w475) -> ("Sync/Reset ACK"=w476:bool)
            n166 = call "Processed_Bytes_To_ES_Packet.vi"("error in (no error)"=w465, "Processed_Bytes"=w462, "ES Packet In"=w463) -> ("error out"=w464:errorcluster, "ES Param Out"=w461:T9)  [unwired: 1 out]
            n167 = Unbundle By Name(w461) -> ("Network Error Status"=w460:T1)
            n168 = Or(x=w477, y=w476) -> (x .or. y?=w459:bool)
            n169 = Or(x=w459, y=w457) -> (x .or. y?=w458:bool)
          }
          n170 = flat-sequence {
            tunnel: w424 -> [w440]
            tunnel: [w440] -> w423
            tunnel: w422 -> [w439]
            tunnel: w418 -> [w438]
            tunnel: [w438] -> w417
            frame #0 {
              n171 = Wait (ms)(milliseconds to wait=w439) -> ()  [unwired: 1 out]
            }
          }
          n172 = Or(x=w420, y=w419) -> (x .or. y?=w421:bool)
          "Try counter (SYNC/RST)" <- w425
        }
      }
    }
  }
  "CM Packet Out" <- w5
  "error out" <- w4
  "CM Params Out" <- w2
  "Network Error Status" <- w1
